vi "LastTDMSfile.vi"(8 "error in (no error)":errorcluster, 11 "Logs Folder":string) -> (0 "error out":errorcluster, 3 "Latest File Saved":string)   [LabVIEW 2011, in "TestStand Library.lvlib"]
uses:
  TestStand Library.lvlib
panel:
  out "All Files in Dir":path[](array[path])
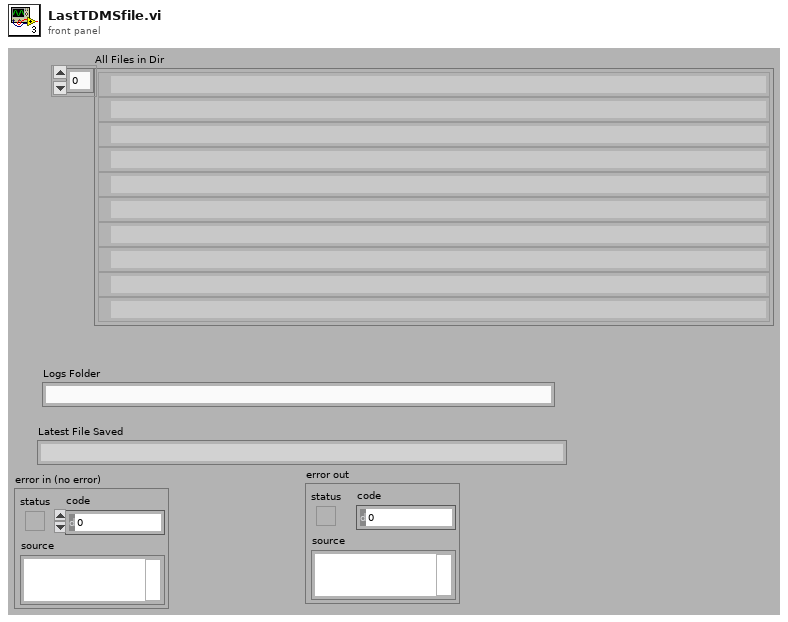
[diagram p1: front panel]
types:
  T1 = cluster{"last mod":timestamp, "file name":path}[]
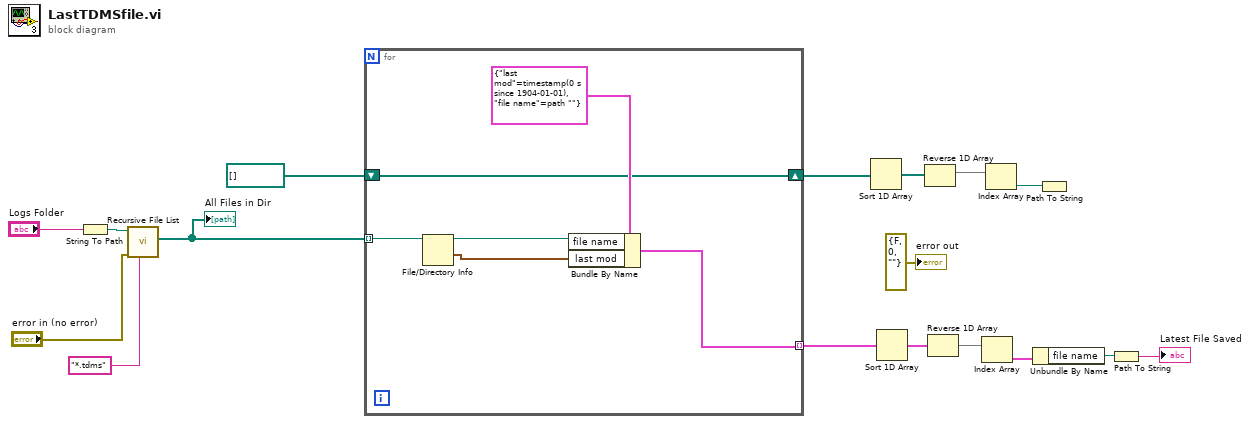
[diagram p0: block diagram]
diagram:
  n1 = String To Path(string="Logs Folder") -> (path=w11:path)
  n2 = call <vilib>:"Recursive File List.vi"("pattern"="*.tdms", "error in (no error)"="error in (no error)", "Folder Path"=w11) -> ("All Files in Dir"=w17:path[])  [unwired: 4 in, 4 out]
  "All Files in Dir" <- w17
  n3 = for {
    tunnel: w17 -> [w23] mode=indexing
    shift-right: [w18] -> w15
    shift-left: path[] [] ("All Files in Dir") -> [w18]
    tunnel: [w19] -> w8 mode=indexing
    n4 = File/Directory Info(path=w23) -> (path out=w21:path, last mod=w20:timestamp)  [unwired: 1 in, 5 out]
    n5 = Bundle By Name(cluster=cluster{"last mod":timestamp, "file name":path} {"last mod"=timestamp(0 s since 1904-01-01), "file name"=path ""}, "file name"=w21, "last mod"=w20) -> (w19:cluster{"last mod":timestamp, "file name":path})
  }
  n6 = Sort 1D Array(array=w15) -> (sorted array=w14:path[])
  n7 = Sort 1D Array(array=w8) -> (sorted array=w7:T1)
  n8 = Reverse 1D Array(array=w14) -> (reversed array=w13:path[])
  n9 = Reverse 1D Array(array=w7) -> (reversed array=w6:T1)
  n10 = Index Array(array=w6) -> (element=w5:cluster{"last mod":timestamp, "file name":path})  [unwired: 1 in]
  n11 = Index Array(array=w13) -> (element=w12:path)  [unwired: 1 in]
  n12 = Unbundle By Name(w5) -> ("file name"=w4:path)
  n13 = Path To String(path=w12) -> ()  [unwired: 1 out]
  n14 = Path To String(path=w4) -> (string=→"Latest File Saved":string)
  "error out" <- errorcluster {"status"=FALSE, "code"=0, "source"=""} ("error out")
